vi "Extract Template Array.vi"(8 "error in (no error)":errorcluster, 11 "vi ref":refnum<vi>) -> (0 "error out":errorcluster, 1 "Found?":bool, 2 "Scripter Input Ref":refnum<vi>, 3 "vi ref out":refnum<vi>)   [LabVIEW 2021]
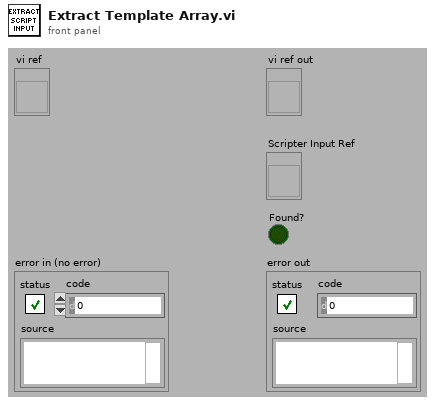
[diagram p1: front panel]
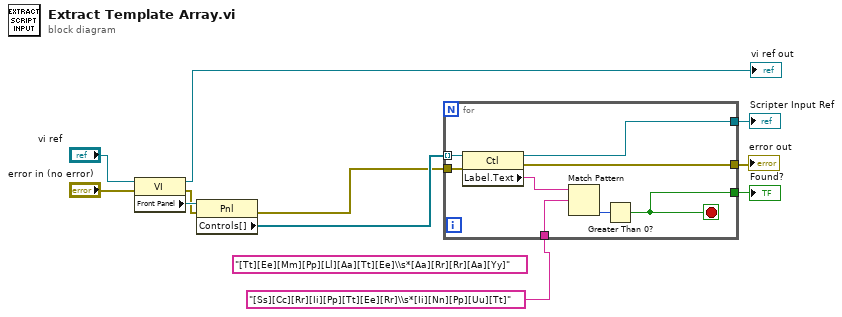
[diagram p0: block diagram]
diagram:
  (unwired) "[Tt][Ee][Mm][Pp][Ll][Aa][Tt][Ee]\\s*[Aa][Rr][Rr][Aa][Yy]" ("regular expression")
  n1 = property class="VI"(reference="vi ref", error in="error in (no error)") -> (reference out=→"vi ref out":refnum<vi>, error out=w5:errorcluster, "Front Panel"=w10:refnum<vi>)
  n2 = property class="Pnl"(reference=w10, error in=w5) -> (error out=w4:errorcluster, "Controls[]"=w11:refnum<vi>[])  [unwired: 1 out]
  n3 = for {
    tunnel: w11 -> [w17] mode=indexing
    tunnel: "[Ss][Cc][Rr][Ii][Pp][Tt][Ee][Rr]\\s*[Ii][Nn][Pp][Uu][Tt]" ("regular expression") -> [w16]
    tunnel: [w15] -> w8
    tunnel: [w14] -> w7
    tunnel: w4 -> [w13]
    tunnel: [w12] -> w3
    stop <- w14 stop-if-true
    n4 = property class="Ctl"(reference=w17, error in=w13) -> (reference out=w15:refnum<vi>, error out=w12:errorcluster, "Label.Text"=w19:string)
    n5 = Match Pattern(string=w19, regular expression=w16) -> (offset past match=w18:i32)  [unwired: 1 in, 3 out]
    n6 = Greater Than 0?(x=w18) -> (x > 0?=w14:bool)
  }
  "error out" <- w3
  "Scripter Input Ref" <- w8
  "Found?" <- w7
